vi "VacuumControlExample.vi"(0 "Vacuum Sensors":T3={"TP On"=FALSE, "IG1 On"=TRUE, "IG2On"=FALSE, "IG Vac Level"=7.206095277894153e-07, "CG1 Vac Level"=7.188197481794052e-05, "CG2 Vac Level"=7.698533430214743e-05, "IG Status"=TRUE} {"CG2 Vac Level" format="%#_2e"; "CG1 Vac Level" format="%#_2e"; "IG Vac Level" format="%#_2e"}, 1 "Gate Valve IG Threshold":dbl=9.9e-06 min=1e-10 max=0.0001, 3 "Charge Step":T4(ring), 5 "Cryo Thresh":dbl, 6 "Turbo Gate":bool=TRUE, 7 "Turbo IG Thresh":dbl=9.9e-06 min=1e-10 max=0.0001, 9 "Cryo 1 Gate":bool=TRUE, 11 "Cryo 2 Gate":bool=TRUE, 12 "Charge Cycle Done":bool caption="Charge\nDone", 13 "Running  \nShot \nSequence":bool, 14 "Puff High\nRef Shot":bool) -> (4 "Cryo 1 Ctrl":bool, 10 "Cryo 2 Ctrl":bool, 15 "Turbo Ctrl":bool)   [LabVIEW 2016]
uses:
  VacuumMeasurementControlState.ctl
panel:
  out "In Shot Time Window":bool
  out "IG Pressure Safe For Charging":bool
  in  "Cap Charge IG Threshold":dbl=9.9e-06 min=1e-10 max=0.0001
  in  "IG Select":bool
  out "IG should turn on":bool
  in  "Cryo Gate 2 Control":T1(ring)
  in  "Turn IG back on after shot (s)":dbl format="%#_13g"
  in  "Time Since Shot (s)":dbl format="%#_13g"
  in  "CG Safety Threshold":dbl
  in  "Cryo Gate 1 Control":T1(ring)
  in  "Ion Gauge Control":T2
  in  "Turbo Gate Control":T1(ring)
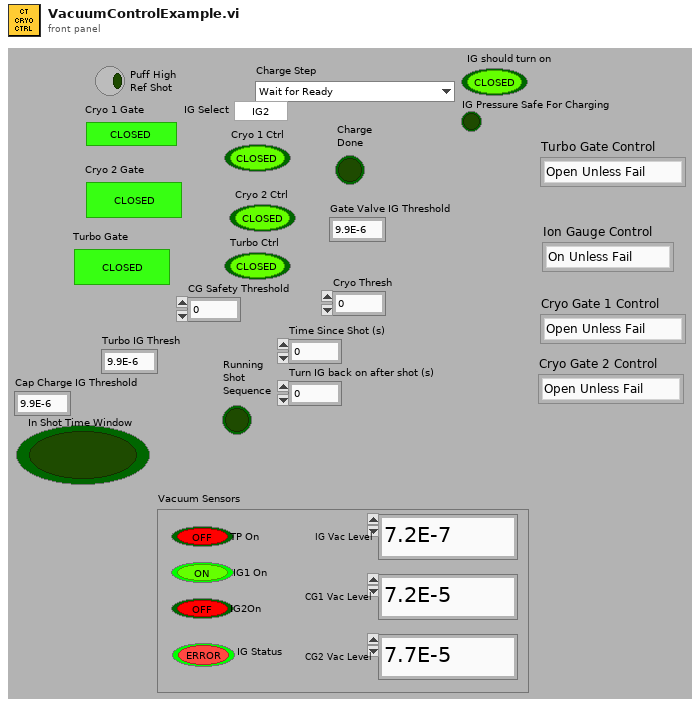
[diagram p1: front panel]
types:
  T1 = enum16{"Open Unless Fail", "Open Unless Shot", "Close"}
  T2 = typedef "VacuumMeasurementControlState.ctl" = enum16{"On Unless Fail", "On Unless Shot", "Force Off", "Manual"}
  T3 = cluster{"TP On":bool, "IG1 On":bool, "IG2On":bool, "IG Vac Level":dbl, "CG1 Vac Level":dbl, "CG2 Vac Level":dbl, "IG Status":bool}
  T4 = enum16{"Wait for Ready", "Prep for Charge", "Open Dump Relays", "Close Connect Relays", "Wait PS Delays", "Wait End of Charge", "Turn Off HV", "Open Connect Relays", "Charge Done"}
  T5 = typedef "VacuumStatus.ctl" = cluster{"Vacuum Sensors":cluster{"TP On":bool, "IG1 On":bool, "IG2On":bool, "IG Vac Level":dbl, "CG1 Vac Level":dbl, "CG2 Vac Level":dbl, "IG Status":bool}, "In Shot Time Window":bool, "IG reading meaningful":bool}
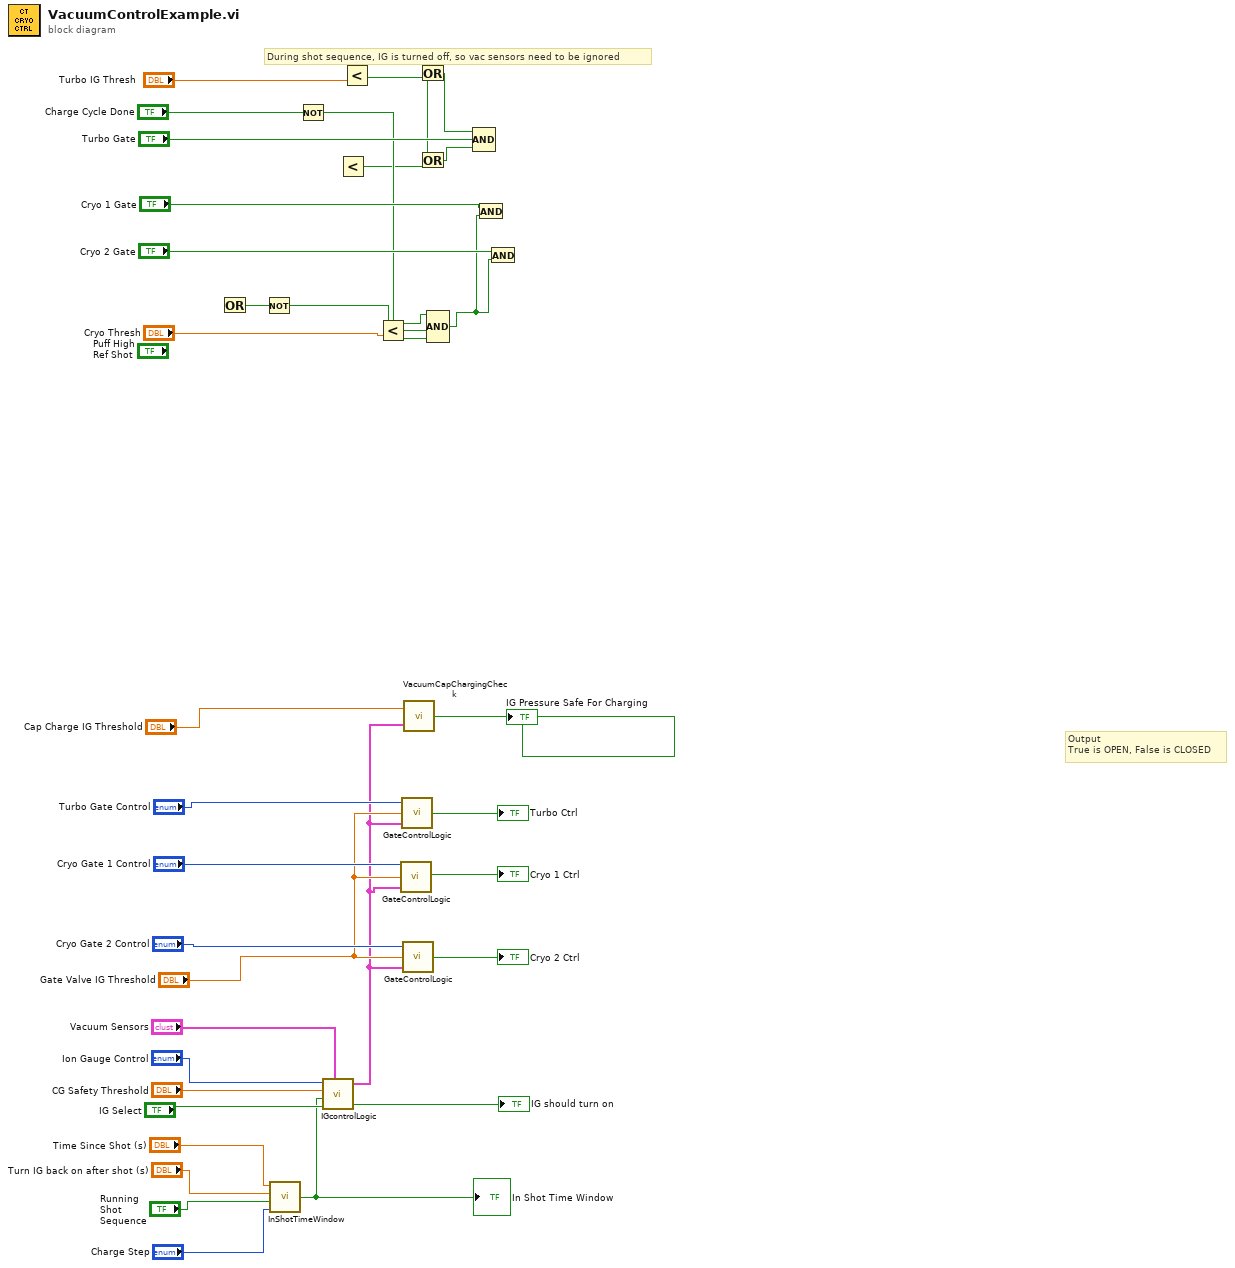
[diagram p0: block diagram]
diagram:
  # "During shot sequence, IG is turned off, so vac sensors need to be ignored"
  # "Output\nTrue is OPEN, False is CLOSED"
  n1 = Or() -> (x .or. y?=w33:bool)  [unwired: 2 in]
  n2 = Not(x=w33) -> (.not. x?=w29:bool)
  n3 = call "InShotTimeWindow.vi"("Charge Step"="Charge Step", "Running  \nShot \nSequence"="Running  \nShot \nSequence", "Turn IG back on after shot (s)"="Turn IG back on after shot (s)", "Time Since Shot (s)"="Time Since Shot (s)") -> ("In Shot Time Window"=w5:bool)
  "In Shot Time Window" <- w5
  n4 = Not(x="Charge Cycle Done") -> (.not. x?=w27:bool)
  n5 = call "IGcontrolLogic.vi"("Ion Gauge Control"="Ion Gauge Control", "CG Safety Threshold"="CG Safety Threshold", "In shot time window"=w5, "IG Select"="IG Select", "Vacuum Sensors"="Vacuum Sensors") -> ("Vacuum Status"=w1:T5, "IG should turn on"=→"IG should turn on":bool)  [unwired: 1 out]
  n6 = Less?() -> (x < y?=w23:bool)  [unwired: 2 in]
  n7 = Less?(y="Turbo IG Thresh") -> (x < y?=w25:bool)  [unwired: 1 in]
  n8 = Less?(y="Cryo Thresh") -> (x < y?=w28:bool)  [unwired: 1 in]
  n9 = call "GateControlLogic.vi"("Vacuum Status"=w1, "Gate Valve IG Threshold"="Gate Valve IG Threshold", "Gate Control"="Cryo Gate 1 Control") -> ("Open Gate"=→"Cryo 1 Ctrl":bool)
  n10 = call "GateControlLogic.vi"("Vacuum Status"=w1, "Gate Valve IG Threshold"="Gate Valve IG Threshold", "Gate Control"="Turbo Gate Control") -> ("Open Gate"=→"Turbo Ctrl":bool)
  n11 = call "GateControlLogic.vi"("Vacuum Status"=w1, "Gate Valve IG Threshold"="Gate Valve IG Threshold", "Gate Control"="Cryo Gate 2 Control") -> ("Open Gate"=→"Cryo 2 Ctrl":bool)
  n12 = call "VacuumCapChargingCheck.vi"("Vacuum Status"=w1, "Cap Charge IG Threshold"="Cap Charge IG Threshold") -> ("IG Pressure Safe For Charging"=→"IG Pressure Safe For Charging":bool)
  n13 = Or(y=w25) -> (x=w21:bool, x .or. y?=w24:bool)
  n14 = Or(x=w21, y=w23) -> (x .or. y?=w22:bool)
  n15 = Compound Arithmetic op=AND(w29, w28, w27) -> (w30:bool)  [unwired: 1 in]
  n16 = Compound Arithmetic op=AND(w24, "Turbo Gate", w22) -> ()  [unwired: 1 out]
  n17 = And(x="Cryo 1 Gate", y=w30) -> ()  [unwired: 1 out]
  n18 = And(x="Cryo 2 Gate", y=w30) -> ()  [unwired: 1 out]
